vi "PH_Synchrolock_Watch.ProcCases.vi"(0 "i ref in":refnum<vi>, 1 "selector":string, 2 "Data":T1, 3 "call cluster":T2={"Object"="", "Selector"="", "CallType"=enum."synchronous", "Async Object"="", "Async Selector"="", "Data Descriptor"="", "Data"=[], "Error #"=0, "Expire"=0}, 5 "error in (no error)":errorcluster) -> (14 "i ref out":refnum<vi>, 17 "answer cluster":T2={"Object"="", "Selector"="", "CallType"=enum."synchronous", "Async Object"="", "Async Selector"="", "Data Descriptor"="", "Data"=[], "Error #"=0, "Expire"=0}, 19 "error out":errorcluster)   [LabVIEW 2014, in "PH_Synchrolock_Watch.lvlib"]
doc: "This method is called by a process from within the default case in the event loop. The methods of a class that are linked to events will be called from THIS method. Add your code here."
uses:
  PH_Synchrolock_Watch.lvlib
  CS_Core/CSSystem/CoreDefs/CoreDefs.call_type.ctl
  CS_Core/BaseProcess/BaseProcess.descriptor string definition.ctl
  CS_Core/CSSystem/CoreDefs/CoreDefs.rawDataType.ctl
  PH_Basics/PH_StatusHandler/PH_StatusHandler.Status.ctl
  CS_Core/CSSystem/CoreLib/CoreLib.string 2 byte array.vi
  CS_Core/CSSystem/CoreLib/CoreLib.byte array 2 int.vi
  CS_Core/CSSystem/CoreLib/CoreLib.byte array 2 short.vi
  CS_Core/CSSystem/CoreLib/CoreLib.byte array 2 double.vi
  CS_Core/BaseProcess/BaseProcess.lvlib
  CS_Core/CSSystem/CoreLib/CoreLib.lvlib
  CS_Core/CAEObj/CAEObj.lvlib
  PH_Basics/PH_PSDBWriter/PH_PSDBWriter.lvlib
  PH_Devices/PH_TKTDS-30xx/PH_TKTDS-30xx.lvlib
  PH_Basics/PH_StatusHandler/PH_StatusHandler.lvlib
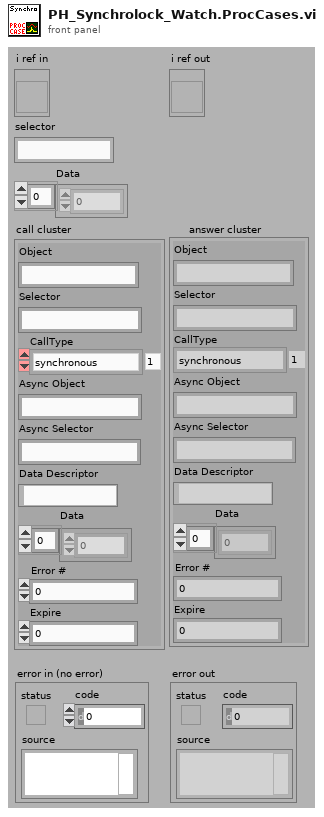
[diagram p1: front panel]
types:
  T1 = typedef "CoreDefs.rawDataType.ctl" = i8[]
  T2 = typedef "CoreDefs.call_type.ctl" = cluster{"Object":string, "Selector":string, "CallType":enum16{"simple", "synchronous", "asynchronous"}, "Async Object":string, "Async Selector":string, "Data Descriptor":T3, "Data":T1, "Error #":i32, "Expire":u32}
  T3 = typedef "BaseProcess.lvlib/BaseProcess.descriptor string definition.ctl" = string
  T4 = typedef "PH_StatusHandler.lvlib/PH_StatusHandler.Status.ctl" = i16
  T5 = typedef "PH_PSDBWriter.lvlib/PH_PSDBWriter.PHELIX-Subsystems.ctl" = i32
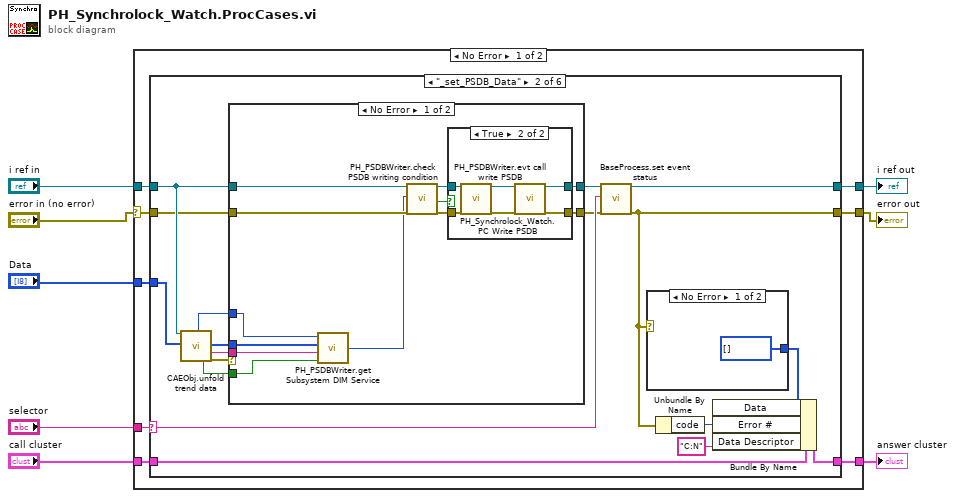
[diagram p0: block diagram]
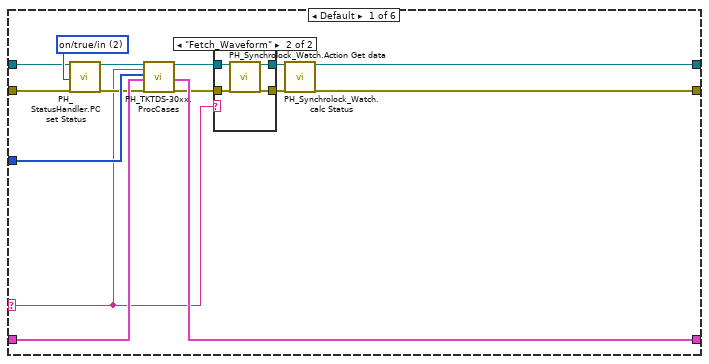
[diagram p2: hidden frame]
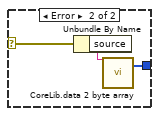
[diagram p6: hidden frame]
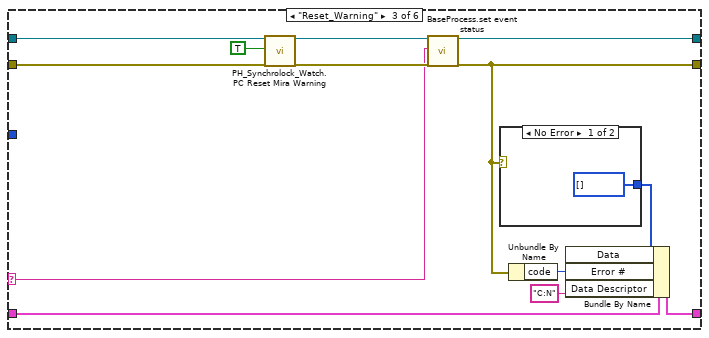
[diagram p7: hidden frame]
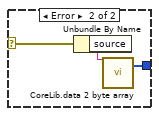
[diagram p8: hidden frame]
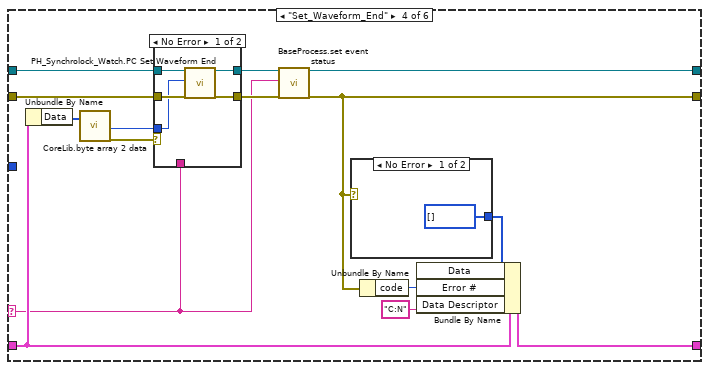
[diagram p9: hidden frame]
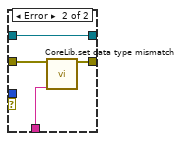
[diagram p10: hidden frame]
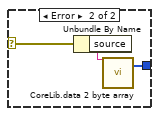
[diagram p11: hidden frame]
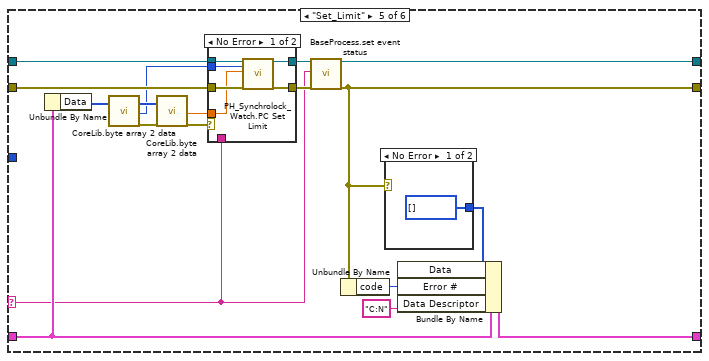
[diagram p12: hidden frame]
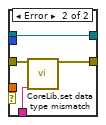
[diagram p13: hidden frame]
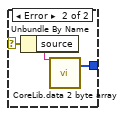
[diagram p14: hidden frame]
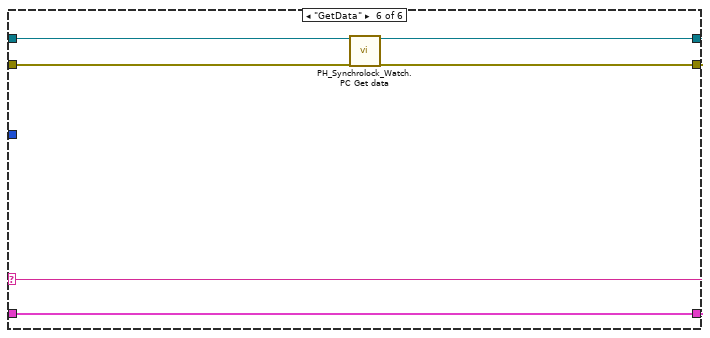
[diagram p15: hidden frame]
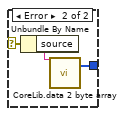
[diagram p16: hidden frame]
diagram:
  n1 = case shown="No Error" "error in (no error)" {
    selector: "error in (no error)" -> [w9 w175]
    tunnel: "selector" -> [w16 _]
    tunnel: [w15 w176] -> w7
    tunnel: "Data" -> [w14 _]
    tunnel: "call cluster" -> [w13 w176]
    tunnel: "i ref in" -> [w12 w177]
    tunnel: [w11 w177] -> w3
    tunnel: [w10 w175] -> w2
    frame No Error {
      n2 = case shown="\"_set_PSDB_Data\"" w16 {
        selector: w16 -> [w17 w50 w83 w100 w132 w164]
        tunnel: w14 -> [w29 w38 _ _ _ _]
        tunnel: w12 -> [w27 w42 w87 w104 w137 w162]
        tunnel: [w23 w49 w90 w109 w140 w166] -> w11
        tunnel: w13 -> [w30 w54 w86 w103 w133 w163]
        tunnel: [w31 w53 w93 w112 w143 w169] -> w15
        tunnel: w9 -> [w25 w40 w88 w105 w136 w161]
        tunnel: [w22 w51 w91 w110 w141 w167] -> w10
        frame Default {
          w28 = T4 2 items=["no info", "off/false/out", "on/true/in", "Failure", "Alarm", "Status 1", "Status 2", "Status 3"] ("Status")
          n3 = call "PH_StatusHandler.PC set Status.vi"("i ref in"=w27, "Status"=w28, "error in (no error)"=w25) -> ("i ref out"=w26:refnum<vi>, "error out"=w24:errorcluster)  [unwired: 15 in]
          n4 = call "PH_TKTDS-30xx.ProcCases.vi"("i ref in"=w26, "selector"=w17, "Data"=w29, "call cluster"=w30, "error in (no error)"=w24) -> ("i ref out"=w21:refnum<vi>, "answer cluster"=w31:T2, "error out"=w19:errorcluster)  [unwired: 12 in]
          n5 = case shown="\"Fetch_Waveform\"" w17 {
            tunnel: w21 -> [w33 w37]
            tunnel: [w33 w36] -> w20
            tunnel: w19 -> [w32 w35]
            tunnel: [w32 w34] -> w18
            frame Default {
            }
            frame "Fetch_Waveform" {
              n6 = call "PH_Synchrolock_Watch.Action Get data.vi"("i ref in"=w37, "error IO"=w35) -> ("i ref out"=w36:refnum<vi>, "error out"=w34:errorcluster)  [unwired: 16 in]
            }
          }
          n7 = call "PH_Synchrolock_Watch.calc Status.vi"("i ref in"=w20, "error in"=w18) -> ("i ref out"=w23:refnum<vi>, "error out"=w22:errorcluster)  [unwired: 16 in]
        }
        frame "_set_PSDB_Data" {
          n8 = call "CAEObj.unfold trend data.vi"("i ref in"=w42, "raw trend data"=w38) -> ("quality"=w43:i32, "no link"=w46:bool, "data"=w44:i8[], "typeDescriptor"=w45:string, "error out"=w47:errorcluster)  [unwired: 9 in, 4 out]
          n9 = case shown="No Error" w47 {
            tunnel: w40 -> [w67 w77]
            tunnel: [w66 w76] -> w41
            tunnel: [w65 w77] -> w39
            tunnel: w42 -> [w63 w76]
            tunnel: w46 -> [w58 _]
            tunnel: w45 -> [w59 _]
            tunnel: w44 -> [w60 _]
            tunnel: w43 -> [w57 _]
            frame No Error {
              n10 = call "PH_PSDBWriter.get Subsystem DIM Service.vi"("no link"=w58, "typeDescriptor"=w59, "data"=w60, "quality"=w57) -> ("PHELIX Subsystems"=w56:T5)
              n11 = call "PH_PSDBWriter.check PSDB writing condition.vi"("i ref in"=w63, "wanted Subsystem"=w56, "error IO"=w67) -> ("i ref out"=w62:refnum<vi>, "write PSDB?"=w61:bool, "error out"=w64:errorcluster)  [unwired: 14 in]
              n12 = case shown="True" w61 {
                tunnel: w64 -> [w68 w75]
                tunnel: [w69 w72] -> w66
                tunnel: [w68 w70] -> w65
                tunnel: w62 -> [w69 w74]
                frame False {
                }
                frame True {
                  n13 = call "PH_Synchrolock_Watch.PC Write PSDB.vi"("i ref in"=w74, "error IO"=w75) -> ("i ref out"=w73:refnum<vi>, "error out"=w71:errorcluster)  [unwired: 16 in]
                  n14 = call "PH_PSDBWriter.evt call write PSDB.vi"("i ref in"=w73, "error in (no error)"=w71) -> ("i ref out"=w72:refnum<vi>, "error out"=w70:errorcluster)  [unwired: 16 in]
                }
              }
            }
            frame Error {
            }
          }
          n15 = call "BaseProcess.set event status.vi"("i ref in"=w41, "EventStatus"=w50, "error in (no error)"=w39) -> ("i ref out"=w49:refnum<vi>, "error out"=w51:errorcluster)  [unwired: 14 in, 1 out]
          n16 = case shown="No Error" w51 {
            selector: w51 -> [_ w81]
            tunnel: [T1 [] ("byteArray out") w80] -> w52
            frame No Error {
            }
            frame Error {
              n17 = Unbundle By Name(w81) -> ("source"=w79:string)
              n18 = call-poly "CoreLib.data 2 byte array.vi"("string"=w79) -> ("byteArray out"=w80:T1)  [unwired: 18 in]
            }
          }
          n19 = Unbundle By Name(w51) -> ("code"=w55:i32)
          n20 = Bundle By Name(cluster=w54, "Data"=w52, "Error #"=w55, "Data Descriptor"="C:N") -> (w53:T2)
        }
        frame "Reset_Warning" {
          n21 = call "PH_Synchrolock_Watch.PC Reset Mira Warning.vi"("i ref in"=w87, "Reset Warning?"=TRUE, "error in (no error)"=w88) -> ("i ref out"=w85:refnum<vi>, "error out"=w84:errorcluster)  [unwired: 15 in]
          n22 = call "BaseProcess.set event status.vi"("i ref in"=w85, "EventStatus"=w83, "error in (no error)"=w84) -> ("i ref out"=w90:refnum<vi>, "error out"=w91:errorcluster)  [unwired: 14 in, 1 out]
          n23 = case shown="No Error" w91 {
            selector: w91 -> [_ w98]
            tunnel: [T1 [] ("byteArray out") w97] -> w92
            frame No Error {
            }
            frame Error {
              n24 = Unbundle By Name(w98) -> ("source"=w96:string)
              n25 = call-poly "CoreLib.data 2 byte array.vi"("string"=w96) -> ("byteArray out"=w97:T1)  [unwired: 18 in]
            }
          }
          n26 = Unbundle By Name(w91) -> ("code"=w94:i32)
          n27 = Bundle By Name(cluster=w86, "Data"=w92, "Error #"=w94, "Data Descriptor"="C:N") -> (w93:T2)
        }
        frame "Set_Waveform_End" {
          n28 = Unbundle By Name(w103) -> ("Data"=w106:T1)
          n29 = call-poly "CoreLib.byte array 2 data.vi"("byteArray"=w106) -> ("i32"=w99:i32, "error out"=w107:errorcluster)  [unwired: 16 in, 1 out]
          n30 = case shown="No Error" w107 {
            tunnel: [w115 w122] -> w102
            tunnel: w104 -> [w117 w122]
            tunnel: w105 -> [w116 w121]
            tunnel: [w118 w120] -> w101
            tunnel: w100 -> [_ w119]
            tunnel: w99 -> [w114 _]
            frame No Error {
              n31 = call "PH_Synchrolock_Watch.PC Set Waveform End.vi"("i ref in"=w117, "Waveform End"=w114, "error in (no error)"=w116) -> ("i ref out"=w115:refnum<vi>, "error out"=w118:errorcluster)  [unwired: 15 in]
            }
            frame Error {
              n32 = call "CoreLib.set data type mismatch.vi"("error in (no error)"=w121, "error source"=w119) -> ("error out"=w120:errorcluster)  [unwired: 17 in]
            }
          }
          n33 = call "BaseProcess.set event status.vi"("i ref in"=w102, "EventStatus"=w100, "error in (no error)"=w101) -> ("i ref out"=w109:refnum<vi>, "error out"=w110:errorcluster)  [unwired: 14 in, 1 out]
          n34 = case shown="No Error" w110 {
            selector: w110 -> [_ w126]
            tunnel: [T1 [] ("byteArray out") w125] -> w111
            frame No Error {
            }
            frame Error {
              n35 = Unbundle By Name(w126) -> ("source"=w124:string)
              n36 = call-poly "CoreLib.data 2 byte array.vi"("string"=w124) -> ("byteArray out"=w125:T1)  [unwired: 18 in]
            }
          }
          n37 = Unbundle By Name(w110) -> ("code"=w113:i32)
          n38 = Bundle By Name(cluster=w103, "Data"=w111, "Error #"=w113, "Data Descriptor"="C:N") -> (w112:T2)
        }
        frame "Set_Limit" {
          n39 = Unbundle By Name(w133) -> ("Data"=w131:T1)
          n40 = call-poly "CoreLib.byte array 2 data.vi"("byteArray"=w131) -> ("byteArray out"=w129:T1, "i16"=w127:i16, "error out"=w130:errorcluster)  [unwired: 16 in]
          n41 = call-poly "CoreLib.byte array 2 data.vi"("byteArray"=w129, "error in (no error)"=w130) -> ("d64"=w138:dbl, "error out"=w128:errorcluster)  [unwired: 15 in, 1 out]
          n42 = case shown="No Error" w128 {
            tunnel: w137 -> [w150 w154]
            tunnel: [w147 w152] -> w134
            tunnel: [w149 w154] -> w135
            tunnel: w138 -> [w145 _]
            tunnel: w132 -> [_ w153]
            tunnel: w136 -> [w148 w151]
            tunnel: w127 -> [w146 _]
            frame No Error {
              n43 = call "PH_Synchrolock_Watch.PC Set Limit.vi"("i ref in"=w150, "Limit to set"=w146, "Limit"=w145, "error in"=w148) -> ("i ref out"=w149:refnum<vi>, "error out"=w147:errorcluster)  [unwired: 14 in]
            }
            frame Error {
              n44 = call "CoreLib.set data type mismatch.vi"("error in (no error)"=w151, "error source"=w153) -> ("error out"=w152:errorcluster)  [unwired: 17 in]
            }
          }
          n45 = call "BaseProcess.set event status.vi"("i ref in"=w135, "EventStatus"=w132, "error in (no error)"=w134) -> ("i ref out"=w140:refnum<vi>, "error out"=w141:errorcluster)  [unwired: 14 in, 1 out]
          n46 = Unbundle By Name(w141) -> ("code"=w144:i32)
          n47 = case shown="No Error" w141 {
            selector: w141 -> [_ w158]
            tunnel: [T1 [] ("byteArray out") w157] -> w142
            frame No Error {
            }
            frame Error {
              n48 = Unbundle By Name(w158) -> ("source"=w156:string)
              n49 = call-poly "CoreLib.data 2 byte array.vi"("string"=w156) -> ("byteArray out"=w157:T1)  [unwired: 18 in]
            }
          }
          n50 = Bundle By Name(cluster=w133, "Data"=w142, "Error #"=w144, "Data Descriptor"="C:N") -> (w143:T2)
        }
        frame "GetData" {
          n51 = call "PH_Synchrolock_Watch.PC Get data.vi"("i ref in"=w162, "error IO"=w161) -> ("i ref out"=w160:refnum<vi>, "error out"=w159:errorcluster)  [unwired: 16 in]
          n52 = call "BaseProcess.set event status.vi"("i ref in"=w160, "EventStatus"=w164, "error in (no error)"=w159) -> ("i ref out"=w166:refnum<vi>, "error out"=w167:errorcluster)  [unwired: 14 in, 1 out]
          n53 = Unbundle By Name(w167) -> ("code"=w170:i32)
          n54 = case shown="No Error" w167 {
            selector: w167 -> [_ w174]
            tunnel: [T1 [] ("byteArray out") w173] -> w168
            frame No Error {
            }
            frame Error {
              n55 = Unbundle By Name(w174) -> ("source"=w172:string)
              n56 = call-poly "CoreLib.data 2 byte array.vi"("string"=w172) -> ("byteArray out"=w173:T1)  [unwired: 18 in]
            }
          }
          n57 = Bundle By Name(cluster=w163, "Data"=w168, "Error #"=w170, "Data Descriptor"="C:N") -> (w169:T2)
        }
      }
    }
    frame Error {
    }
  }
  "answer cluster" <- w7
  "i ref out" <- w3
  "error out" <- w2
